vi "Verify Chan Volt Cal Test one channel at a time.vi"(8 "error in (no error)":errorcluster, 9 "nScale":i32, 11 "nWhichChan":i32) -> (0 "error out":errorcluster, 3 "Channel Voltage Result":dbl)   [LabVIEW 2013]
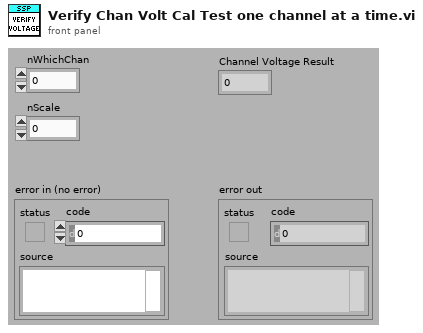
[diagram p1: front panel]
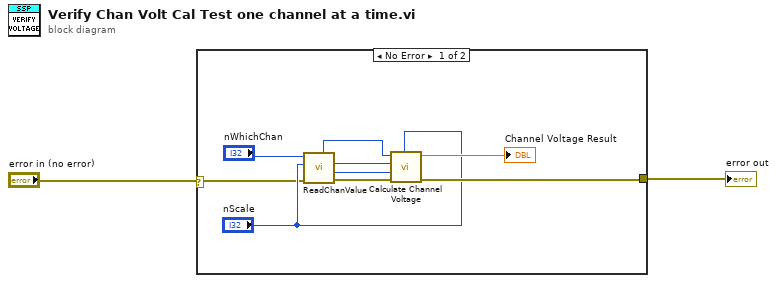
[diagram p0: block diagram]
diagram:
  n1 = case shown="No Error" "error in (no error)" {
    selector: "error in (no error)" -> [w3 w12]
    tunnel: [w6 w12] -> w2
    frame No Error {
      n2 = call "ReadChanValue.vi"("error in (no error)"=w3, "nScale"="nScale", "nWhichChan"="nWhichChan") -> ("error out"=w11:errorcluster, "*pnChanSpanOffset"=w8:i32, "*pnChanZeroOffset"=w9:i32, "*pnChanValue"=w10:i32)  [unwired: 4 in, 1 out]
      n3 = call "Calculate Channel Voltage.vi"("Scale"="nScale", "error in (no error)"=w11, "ChanSpanOffset"=w8, "ChanZeroOffset"=w9, "ChanValue"=w10) -> ("error out"=w6:errorcluster, "Channel Voltage Result"=→"Channel Voltage Result":dbl)  [unwired: 5 in]
    }
    frame Error {
    }
  }
  "error out" <- w2
